vi "Detach GUI Controls.vi"(8 "error in (no error)":errorcluster, 10 "GUI Control":refnum<class "GUI Control.lvclass">, 11 "Panel GUI Manager in":refnum<class "Panel GUI Manager.lvclass">) -> (0 "error out":errorcluster, 3 "Panel GUI Manager out":refnum<class "Panel GUI Manager.lvclass">)   [LabVIEW 2015, in "Panel GUI Manager.lvclass"]
uses:
  Panel GUI Manager.lvclass
  GUI/GUI Controls/GUI Control/GUI Control.lvclass
  Panel GUI Manager.lvclass/Panel GUI Manager.ctl
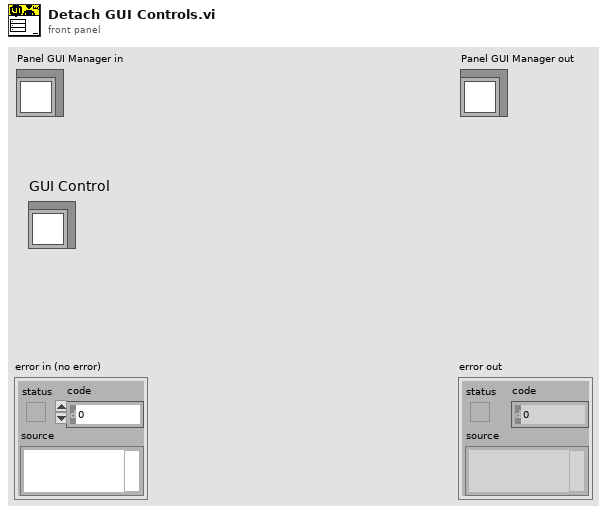
[diagram p1: front panel]
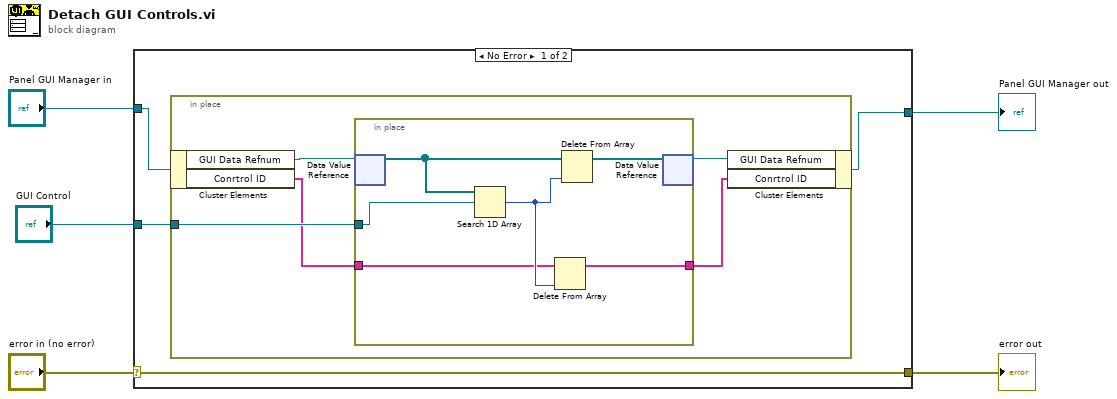
[diagram p0: block diagram]
diagram:
  n1 = case shown="No Error" "error in (no error)" {
    selector: "error in (no error)" -> [w9 w22]
    tunnel: [w9 w22] -> w4
    tunnel: [w6 w21] -> w2
    tunnel: "Panel GUI Manager in" -> [w7 w21]
    tunnel: "GUI Control" -> [w8 _]
    frame No Error {
      n2 = in-place {
        in-place-border: w8 -> [w14]
        n3 = in-place-cluster #1(w7) -> ("GUI Data Refnum"=w13:refnum<data-value>, "Conrtrol ID"=w12:string[])
        n4 = in-place {
          in-place-border: w14 -> [w20]
          in-place-border: w12 -> [w16]
          in-place-border: [w15] -> w11
          n5 = in-place-dvr #2(w13) -> (w19:refnum<class "GUI Control.lvclass">[])  [unwired: 1 out]
          n6 = Search 1D Array(1D array=w19, element=w20) -> (index of element=w17:i32)  [unwired: 1 in]
          n7 = Delete From Array(array=w16, index=w17) -> (array with subset deleted=w15:string[])  [unwired: 1 in, 1 out]
          n8 = Delete From Array(array=w19, index=w17) -> (array with subset deleted=w18:refnum<class "GUI Control.lvclass">[])  [unwired: 1 in, 1 out]
          n9 = in-place-dvr #2(w18) -> (w10:refnum<data-value>)  [unwired: 1 out]
        }
        n10 = in-place-cluster #1("GUI Data Refnum"=w10, "Conrtrol ID"=w11) -> (w6:refnum<class "Panel GUI Manager.lvclass">)
      }
    }
    frame Error {
    }
  }
  "error out" <- w4
  "Panel GUI Manager out" <- w2
